vi "op_x2_Temperatures.vi"(8 "IP address 2":string="172.16.14.23", 9 "ENA2":bool caption="Connection 2 enable", 10 "IP address 1":string="172.16.14.22", 11 "ENA1":bool caption="Connection 1 enable") -> (0 "error out":errorcluster, 1 "values string":string, 2 "T histogram":T1(graph) caption="Temperature histogram", 3 "mean":sgl format="%.1g ºC", 5 "ChipID+T array":u32[](array[numeric]) format="%.0x")   [LabVIEW 2015, in "VIPM2.lvlib"]
doc: "Operation: <b>Read Temperature</b> from 2 FPGAs simultaneously.\nFa dues crides a <b>Get Temperature.vi</b> amb reentrança.\nElimina errors aberrants per estadística i retorna valors.\nInclou LOG de temperatures en arxiu."
uses:
  VIPM2.lvlib
  <vilib>/Analysis/NI_AALBase.lvlib
panel:
  out "bons %":u8
  out "standard deviation":sgl format="%#.1g ºC"
  out "standard deviation raw":sgl format="%#.1g ºC"
  out "mean raw":sgl format="%.1g ºC"
  out "T histogram raw":T1(graph) caption="Temperature histogram"
  # "Operation: Temperature from 2 FPGAs simultaneously"
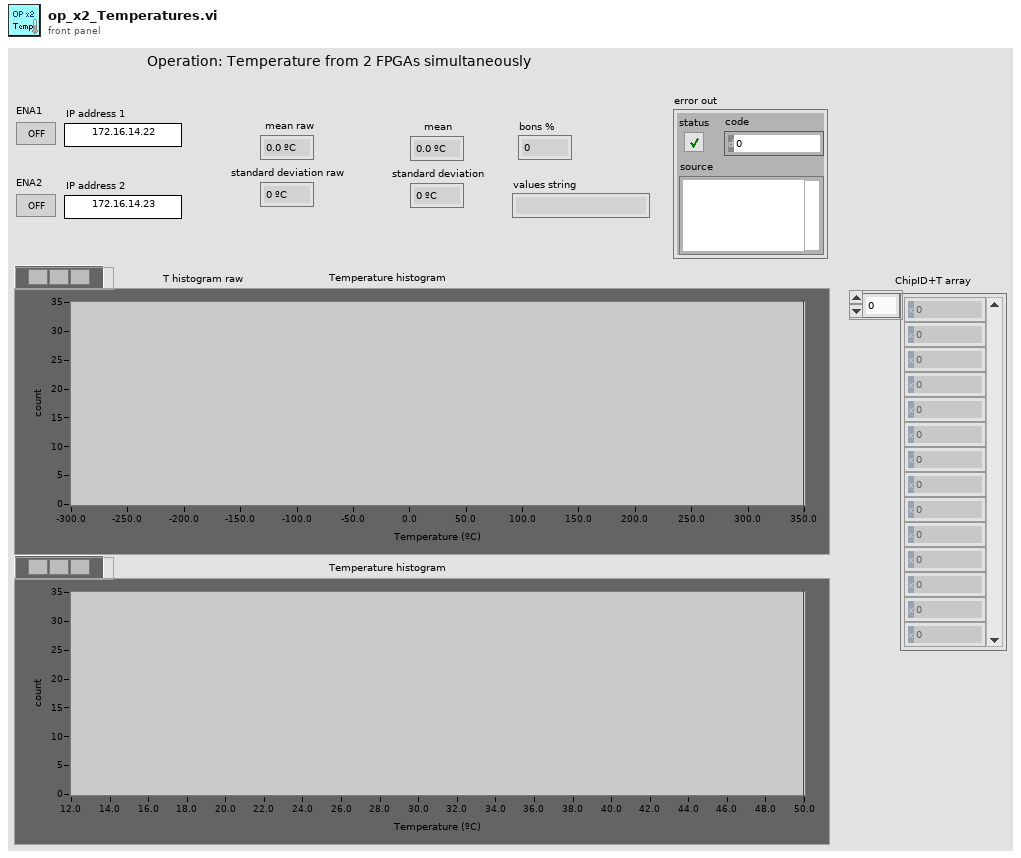
[diagram p1: front panel]
types:
  T1 = cluster{"X Values":dbl[], "Histogram: h(x)":i32[]}
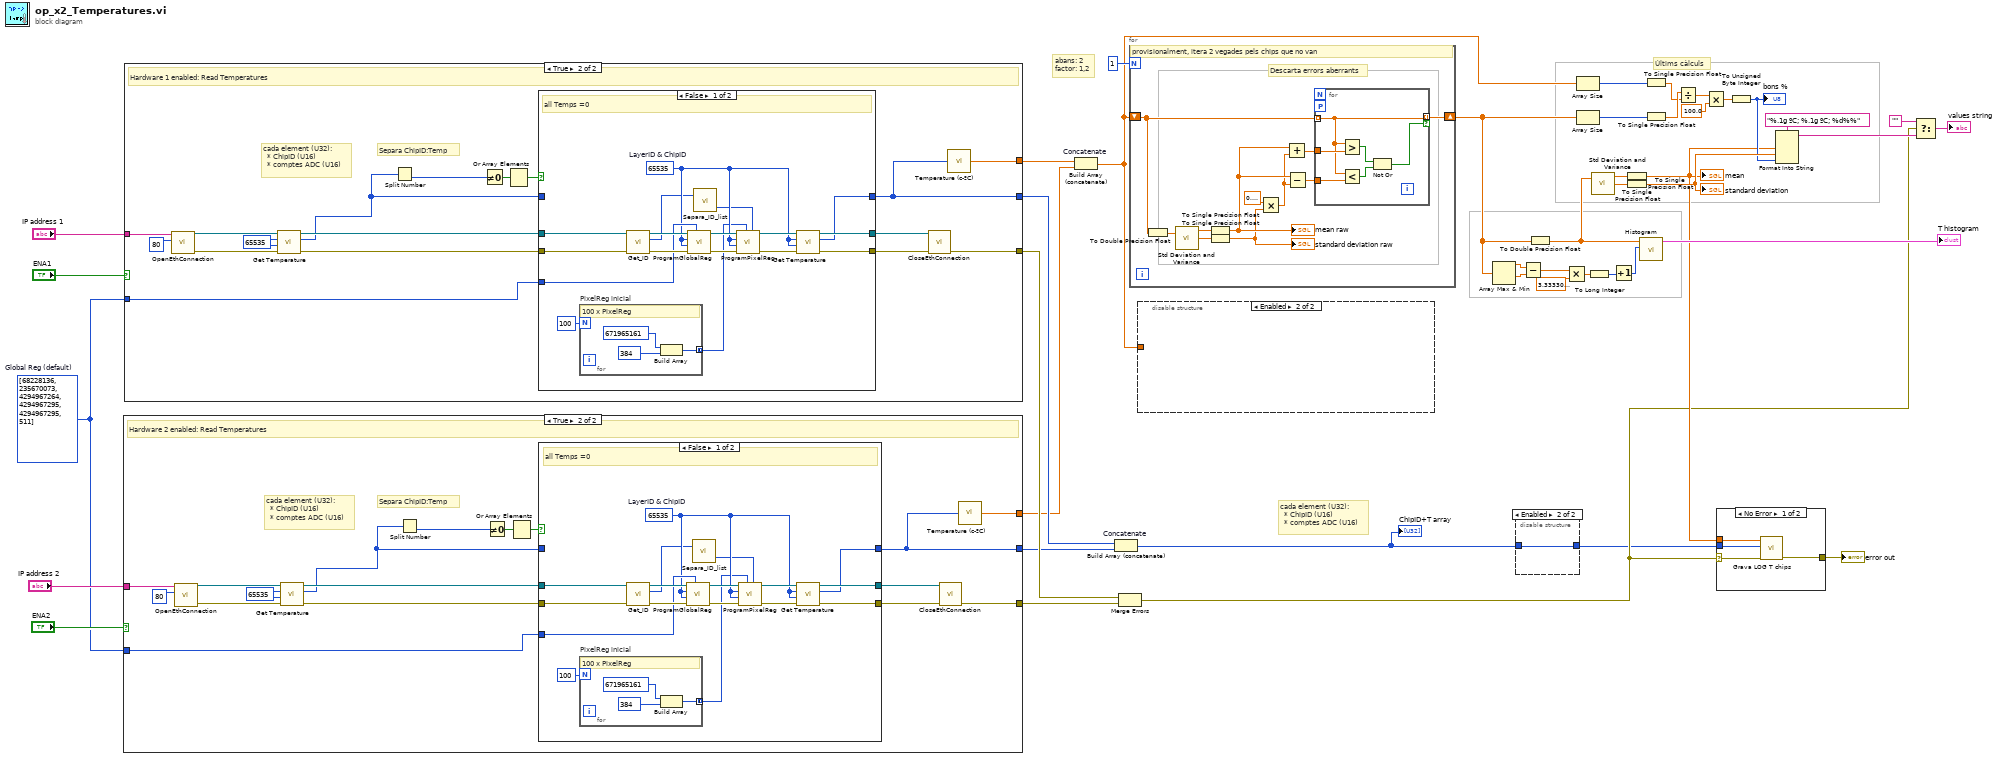
[diagram p0: block diagram]
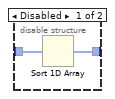
[diagram p6: hidden frame]
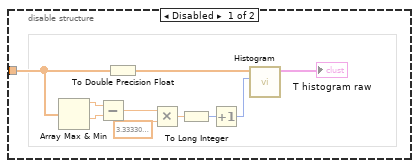
[diagram p8: hidden frame]
diagram:
  w39 = u32[] [68228136, 235670073, 4294967264, 4294967295, 4294967295, 511]  # Global Reg (default)
  # "abans: 2\nfactor: 1,2"
  # "Últims càlculs"
  # "cada element (U32):\n  * ChipID (U16)\n  * comptes ADC (U16)"
  n1 = case shown="True" "ENA2" {
    tunnel: "IP address 2" -> [_ w60]
    tunnel: w39 -> [_ w52]
    tunnel: [_ w49] -> w38
    tunnel: [_ w48] -> w33
    tunnel: [_ w46] -> w36
    frame False {
      # "Hardware 2 not enabled"
    }
    frame True {
      w44 = u32 65535 ("LayerID")
      # "Separa ChipID:Temp"
      # "cada element (U32):\n  * ChipID (U16)\n  * comptes ADC (U16)"
      # "Hardware 2 enabled: Read Temperatures"
      n2 = call "OpenEthConnection.vi"("Port"=u16 80, "IP address"=w60) -> ("error out"=w57:errorcluster, "connection ID out"=w58:refnum<k5>)  [unwired: 7 in, 1 out]
      n3 = call "Get Temperature.vi"("error in (no error)"=w57, "ChipID"=w44, "LayerID"=w44, "connection ID"=w58) -> ("error out"=w53:errorcluster, "Temperatures"=w47:u32[], "connection ID out"=w54:refnum<k5>)  [unwired: 4 in, 1 out]
      n4 = Split Number(x=w47) -> (lo(x)=w45:u16[])  [unwired: 1 out]
      n5 = Not Equal To 0?(x=w45) -> (x != 0?=w56:bool[])
      n6 = Or Array Elements(Boolean array=w56) -> (logical OR=w55:bool)
      n7 = case shown="False" w55 {
        tunnel: w47 -> [_ w81]
        tunnel: [w63 w81] -> w46
        tunnel: [w72 w83] -> w51
        tunnel: w54 -> [w77 w83]
        tunnel: [w71 w82] -> w50
        tunnel: w53 -> [w76 w82]
        tunnel: w52 -> [w73 _]
        frame False {
          w66 = u32 65535  # LayerID & ChipID
          # "all Temps =0"
          n8 = for "PixelReg inicial" {
            N: 100 -> [_]
            tunnel: [w79] -> w61 mode=concatenating
            # "100 x PixelReg"
            n9 = Build Array(u32 671965161 ("Numeric"), u32 384 ("x")) -> (w79:u32[])
          }
          n10 = call "Get_ID.vi"("error in (no error)"=w76, "connection ID"=w77) -> ("error out"=w74:errorcluster, "All ID list"=w65:u32[], "connection ID out"=w75:refnum<k5>)  [unwired: 6 in, 1 out]
          n11 = call "ProgramGlobalReg.vi"("Global Reg"=w73, "error in (no error)"=w74, "ChipID"=w66, "LayerID"=w66, "connection ID"=w75) -> ("error out"=w68:errorcluster, "connection ID out"=w70:refnum<k5>)  [unwired: 2 in, 3 out]
          n12 = call "Separa_ID_list.vi"("All ID list"=w65) -> ("Chip ID list"=w64:u32[])  [unwired: 1 in, 1 out]
          n13 = call "ProgramPixelReg.vi"("Chip ID list"=w64, "Pixel Register"=w61, "error in (no error)"=w68, "ChipID"=w66, "LayerID"=w66, "connection ID"=w70) -> ("error out"=w67:errorcluster, "connection ID out"=w69:refnum<k5>)  [unwired: 1 in, 3 out]
          n14 = call "Get Temperature.vi"("error in (no error)"=w67, "ChipID"=w66, "LayerID"=w66, "connection ID"=w69) -> ("error out"=w71:errorcluster, "Temperatures"=w63:u32[], "connection ID out"=w72:refnum<k5>)  [unwired: 4 in, 1 out]
        }
        frame True {
          # "some Temp <>0"
        }
      }
      n15 = call "CloseEthConnection.vi"("error in (no error)"=w50, "connection ID"=w51) -> ("error out"=w49:errorcluster)  [unwired: 9 in]
      n16 = call "Temperature (c-ºC).vi"("ChipID + Tcounts"=w46) -> ("Temperatures in ºC"=w48:sgl[])  [unwired: 3 in]
    }
  }
  n17 = case shown="True" "ENA1" {
    tunnel: "IP address 1" -> [_ w100]
    tunnel: w39 -> [_ w92]
    tunnel: [_ w89] -> w37
    tunnel: [_ w88] -> w34
    tunnel: [_ w86] -> w35
    frame False {
      # "Hardware 1 not enabled"
    }
    frame True {
      w84 = u32 65535 ("LayerID")
      # "Separa ChipID:Temp"
      # "cada element (U32):\n  * ChipID (U16)\n  * comptes ADC (U16)"
      # "Hardware 1 enabled: Read Temperatures"
      n18 = call "OpenEthConnection.vi"("Port"=u16 80, "IP address"=w100) -> ("error out"=w97:errorcluster, "connection ID out"=w98:refnum<k5>)  [unwired: 7 in, 1 out]
      n19 = call "Get Temperature.vi"("error in (no error)"=w97, "ChipID"=w84, "LayerID"=w84, "connection ID"=w98) -> ("error out"=w93:errorcluster, "Temperatures"=w87:u32[], "connection ID out"=w94:refnum<k5>)  [unwired: 4 in, 1 out]
      n20 = Split Number(x=w87) -> (lo(x)=w85:u16[])  [unwired: 1 out]
      n21 = Not Equal To 0?(x=w85) -> (x != 0?=w96:bool[])
      n22 = Or Array Elements(Boolean array=w96) -> (logical OR=w95:bool)
      n23 = case shown="False" w95 {
        tunnel: w87 -> [_ w123]
        tunnel: [w103 w123] -> w86
        tunnel: [w112 w122] -> w91
        tunnel: w94 -> [w117 w122]
        tunnel: [w111 w121] -> w90
        tunnel: w93 -> [w116 w121]
        tunnel: w92 -> [w113 _]
        frame False {
          w106 = u32 65535  # LayerID & ChipID
          # "all Temps =0"
          n24 = for "PixelReg inicial" {
            N: 100 -> [_]
            tunnel: [w119] -> w101 mode=concatenating
            # "100 x PixelReg"
            n25 = Build Array(u32 671965161 ("Numeric"), u32 384 ("x")) -> (w119:u32[])
          }
          n26 = call "Get_ID.vi"("error in (no error)"=w116, "connection ID"=w117) -> ("error out"=w114:errorcluster, "All ID list"=w105:u32[], "connection ID out"=w115:refnum<k5>)  [unwired: 6 in, 1 out]
          n27 = call "ProgramGlobalReg.vi"("Global Reg"=w113, "error in (no error)"=w114, "ChipID"=w106, "LayerID"=w106, "connection ID"=w115) -> ("error out"=w108:errorcluster, "connection ID out"=w110:refnum<k5>)  [unwired: 2 in, 3 out]
          n28 = call "Separa_ID_list.vi"("All ID list"=w105) -> ("Chip ID list"=w104:u32[])  [unwired: 1 in, 1 out]
          n29 = call "ProgramPixelReg.vi"("Chip ID list"=w104, "Pixel Register"=w101, "error in (no error)"=w108, "ChipID"=w106, "LayerID"=w106, "connection ID"=w110) -> ("error out"=w107:errorcluster, "connection ID out"=w109:refnum<k5>)  [unwired: 1 in, 3 out]
          n30 = call "Get Temperature.vi"("error in (no error)"=w107, "ChipID"=w106, "LayerID"=w106, "connection ID"=w109) -> ("error out"=w111:errorcluster, "Temperatures"=w103:u32[], "connection ID out"=w112:refnum<k5>)  [unwired: 4 in, 1 out]
        }
        frame True {
          # "some Temp <>0"
        }
      }
      n31 = call "CloseEthConnection.vi"("error in (no error)"=w90, "connection ID"=w91) -> ("error out"=w89:errorcluster)  [unwired: 9 in]
      n32 = call "Temperature (c-ºC).vi"("ChipID + Tcounts"=w86) -> ("Temperatures in ºC"=w88:sgl[])  [unwired: 3 in]
    }
  }
  n33 = Build Array (concatenate) "Concatenate"(w34, w33) -> (w8:sgl[])
  n34 = Build Array (concatenate) "Concatenate"(w35, w36) -> (w6:u32[])
  "ChipID+T array" <- w6
  n35 = Merge Errors "Merge Errors"(w37, w38) -> (w11:errorcluster)
  n36 = for {
    N: 1 -> [_]
    shift-right: [w125] -> w10
    shift-left: w8 -> [w124]
    # "Descarta errors aberrants"
    # "provisionalment, itera 2 vegades pels chips que no van"
    n37 = To Double Precision Float(number=w124) -> (double precision float=w129:dbl[])
    n38 = call <vilib>:"Std Deviation and Variance.vi"("X"=w129) -> ("mean"=w134:dbl, "standard deviation"=w133:dbl)  [unwired: 1 in, 1 out]
    n39 = To Single Precision Float(number=w134) -> (single precision float=w132:sgl)
    "mean raw" <- w132
    n40 = To Single Precision Float(number=w133) -> (single precision float=w128:sgl)
    "standard deviation raw" <- w128
    n41 = Multiply(x=sgl 0.8, y=w128) -> (x*y=w127:sgl)
    n42 = Add(x=w132, y=w127) -> (x+y=w131:sgl)
    n43 = Subtract(x=w132, y=w127) -> (x-y=w130:sgl)
    n44 = for {
      tunnel: w131 -> [w140]
      tunnel: w130 -> [w135]
      tunnel: w124 -> [w136] mode=indexing
      tunnel: [w136] -> w125 mode=indexing if=w137
      workers-P: _ -> [_]
      n45 = Greater?(x=w136, y=w140) -> (0:w139:bool)
      n46 = Less?(x=w136, y=w135) -> (x < y?=w138:bool)
      n47 = Not Or(1:w138, 2:w139) -> (0:w137:bool)
    }
  }
  n48 = disable-structure shown="Enabled" {
    disable-tunnel: w8 -> [w147 _]
    frame Disabled {
      n49 = Array Max & Min(array=w147) -> (max value=w149:sgl, min value=w150:sgl)  [unwired: 2 out]
      n50 = Subtract(x=w149, y=w150) -> (x-y=w144:sgl)
      n51 = To Double Precision Float(number=w147) -> (double precision float=w148:dbl[])
      n52 = Multiply(x=w144, y=sgl 3.3333 ("x")) -> (x*y=w142:sgl)
      n53 = To Long Integer(number=w142) -> (32bit integer=w141:i32)
      n54 = Increment(x=w141) -> (x+1=w145:i32)
      n55 = call <vilib>:"Histogram.vi"("intervals"=w145, "X"=w148) -> ("Histogram Graph"=→"T histogram raw":T1)  [unwired: 6 in, 3 out]
    }
    frame Enabled {
    }
  }
  n56 = Array Max & Min(array=w10) -> (max value=w30:sgl, min value=w29:sgl)  [unwired: 2 out]
  n57 = disable-structure shown="Enabled" {
    disable-tunnel: w6 -> [w152 w153]
    disable-tunnel: [w151 w153] -> w5
    frame Disabled {
      n58 = Sort 1D Array(array=w152) -> (sorted array=w151:u32[])
    }
    frame Enabled {
    }
  }
  n59 = Subtract(x=w30, y=w29) -> (x-y=w3:sgl)
  n60 = To Double Precision Float(number=w10) -> (double precision float=w28:dbl[])
  n61 = Multiply(x=w3, y=sgl 3.3333 ("x")) -> (x*y=w2:sgl)
  n62 = Array Size(array=w8) -> (size(s)=w26:i32)
  n63 = Array Size(array=w10) -> (size(s)=w25:i32)
  n64 = To Long Integer(number=w2) -> (32bit integer=w1:i32)
  n65 = call <vilib>:"Std Deviation and Variance.vi"("X"=w28) -> ("mean"=w31:dbl, "standard deviation"=w32:dbl)  [unwired: 1 in, 1 out]
  n66 = Increment(x=w1) -> (x+1=w7:i32)
  n67 = To Single Precision Float(number=w31) -> (single precision float=w16:sgl)
  "mean" <- w16
  n68 = To Single Precision Float(number=w32) -> (single precision float=w18:sgl)
  "standard deviation" <- w18
  n69 = call <vilib>:"Histogram.vi"("intervals"=w7, "X"=w28) -> ("Histogram Graph"=→"T histogram":T1)  [unwired: 6 in, 3 out]
  n70 = To Single Precision Float(number=w26) -> (single precision float=w23:sgl)
  n71 = To Single Precision Float(number=w25) -> (single precision float=w24:sgl)
  n72 = Divide(x=w24, y=w23) -> (x/y=w22:sgl)
  n73 = Multiply(x=w22, y=sgl 100.0) -> (x*y=w20:sgl)
  n74 = case shown="No Error" w11 {
    selector: w11 -> [w154 w158]
    tunnel: w5 -> [w157 _]
    tunnel: w16 -> [w156 _]
    tunnel: [w155 w158] -> w15
    frame No Error {
      n75 = call "Grava LOG T chips.vi"("error in"=w154, "Array ChipID+Temp"=w157, "Temperature mean"=w156) -> ("error out"=w155:errorcluster)  [unwired: 8 in]
    }
    frame Error {
    }
  }
  "error out" <- w15
  n76 = To Unsigned Byte Integer(number=w20) -> (unsigned 8bit integer=w17:u8)
  "bons %" <- w17
  n77 = Format Into String(format string="%.1g ºC; %.1g ºC; %d%%", w16, w18, w17) -> (resulting string=w14:string)  [unwired: 2 in, 1 out]
  n78 = Select(t="", s=w11, f=w14) -> (s? t:f=→"values string":string)
